vi "Set Charge Shifting.vi"(8 "error in (no error)":errorcluster, 10 "NumberRepeats":u32, 11 "NumberRows":u32) -> (0 "error out":errorcluster, 3 "function return":u32)   [LabVIEW 2014, in "atmcd32d.lvlib"]
doc: "unsigned int WINAPI SetChargeShifting(unsigned int NumberRows, unsigned int NumberRepeats);"
uses:
  atmcd32d.lvlib
  atmcd32d.dll
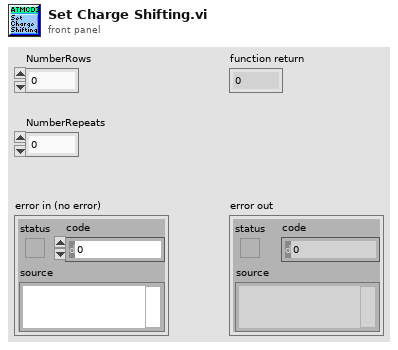
[diagram p1: front panel]
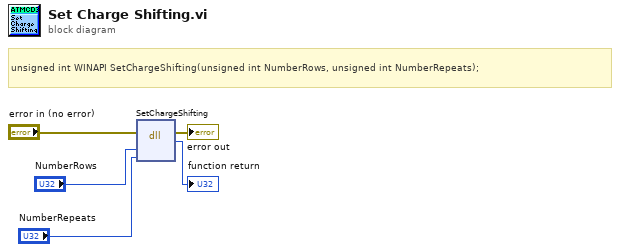
[diagram p0: block diagram]
diagram:
  # "unsigned int WINAPI SetChargeShifting(unsigned int NumberRows, unsigned int NumberRepeats);"
  n1 = dll-call lib="C:/Users/Bakir/Documents/Lambda2-Testing/lib/Andorlib/atmcd32d.*" fn="SetChargeShifting"(error in="error in (no error)", "NumberRows"="NumberRows", "NumberRepeats"="NumberRepeats") -> (error out=→"error out":errorcluster, →"function return":u32)  [unwired: 4 in, 1 out]
